vi "Autonomous Independent.vi"() -> ()   [LabVIEW 2014]
doc: "This VI is called when autonomous begins, and will automatically be terminated when autonomous ends. You can carry out timed or sensor driven robot movement independently without needing to return to the caller."
uses:
  <vilib>/ActorFramework/Message Enqueuer/Message Priority.ctl
  Robot Actor Framework/System Actor/System Actor Messages/Trace Msg/Trace Msg.lvclass/Trace Msg.ctl
  <vilib>/ActorFramework/Message Enqueuer/Message Enqueuer.lvclass/Message Enqueuer.ctl
  <vilib>/ActorFramework/Message Enqueuer/Enqueue.vi
  <vilib>/Utility/config.llb/Read Key (Boolean).vi
  Robot Global Data.vi
  <vilib>/Utility/config.llb/Read Key (U32).vi
  <vilib>/Utility/config.llb/Read Key (Double).vi
  <vilib>/ActorFramework/Message Priority Queue/Priority Enqueue.vi
  Robot/Forward Drive/Forward Drive Messages/Set Percentage Msg/Set Percentage Msg.lvclass
  Robot Actor Framework/System Actor/System Actor Messages/Trace Msg/Trace Msg.lvclass
  <vilib>/Utility/config.llb/NI_LVConfig.lvlib
  <vilib>/ActorFramework/Message Enqueuer/Message Enqueuer.lvclass
panel:
  in  "Time(ms)":u32=2500
  in  "Rate(Percentage)":dbl=-1.0 min=-1.0 max=1.0
  # "Be sure to right-click and choose Data Operations>>Make Current Value default if you want to save the array values with the VI"
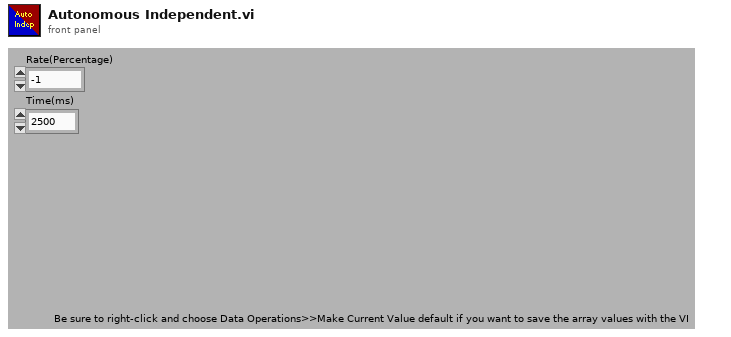
[diagram p1: front panel]
types:
  T1 = typedef "Actor Framework.lvlib/Message Enqueuer.lvclass/Message Priority.ctl" = enum16{"Low", "Normal", "High"}
  T2 = enum16{"Critical", "Error", "Warning", "Informational", "Debug"}
  T3 = typedef "NI_LVConfig.lvlib/Config Data RefNum.ctl" = refnum<k1>
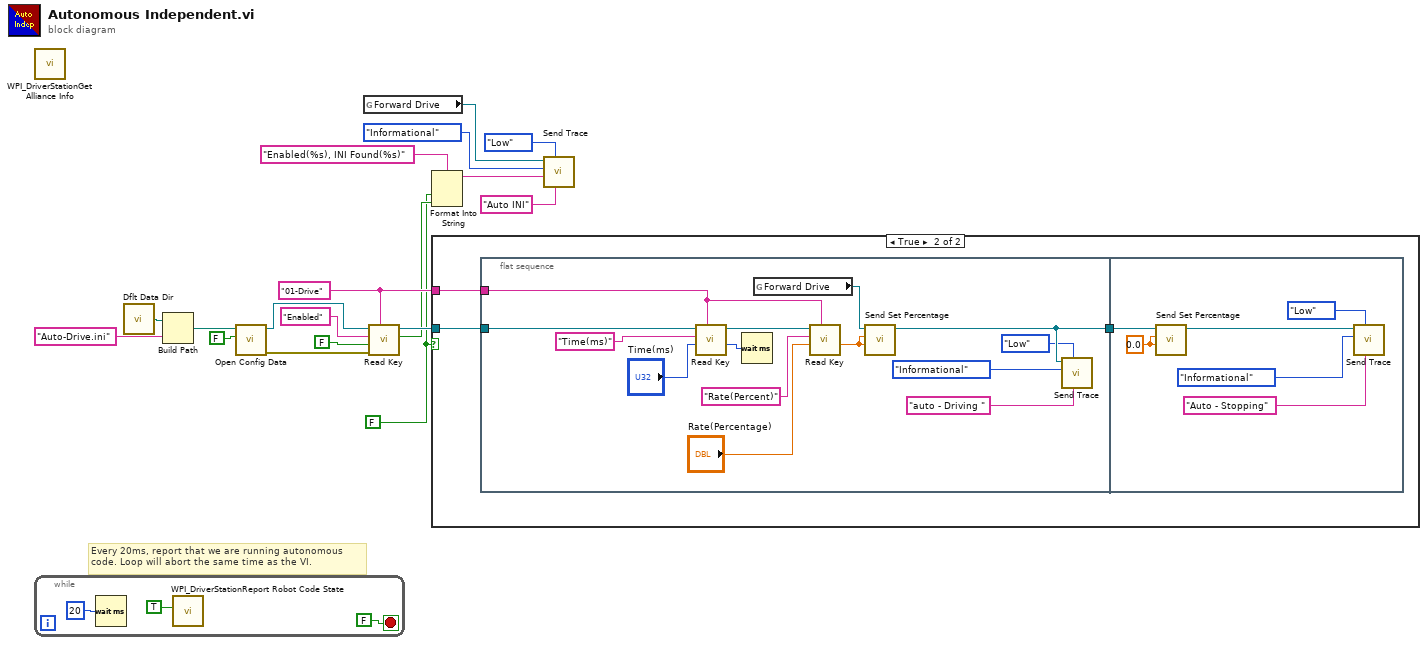
[diagram p0: block diagram]
diagram:
  w1 = FALSE
  w12 = "01-Drive" ("section")
  # "Every 20ms, report that we are running autonomous\ncode. Loop will abort the same time as the VI."
  n1 = call <vilib>:"WPI_DriverStationGet Alliance Info.vi"() -> ()  [unwired: 12 out]
  n2 = while {
    stop <- FALSE stop-if-true
    n3 = Wait (ms)(milliseconds to wait=u32 20) -> ()  [unwired: 1 out]
    n4 = call <vilib>:"WPI_DriverStationReport Robot Code State.vi"("Autonomous"=TRUE) -> ()  [unwired: 10 in, 1 out]
  }
  n5 = call <vilib>:"Dflt Data Dir.vi"() -> ("App:Default Data Directory"=w16:path)
  n6 = Build Path(base path=w16, name or relative path="Auto-Drive.ini" ("text")) -> (appended path=w15:path)
  n7 = call <vilib>:"Open Config Data.vi"("create file if necessary (T)"=FALSE, "configuration file path"=w15) -> ("error out"=w9:errorcluster, "refnum"=w14:T3)  [unwired: 7 in, 1 out]
  n8 = global read "Robot Global Data.vi" "Forward Drive"() -> (w8:refnum<class "Message Enqueuer.lvclass">)
  n9 = call-poly <vilib>:"Read Key.vi"("section"=w12, "error in (no error)"=w9, "default value"=FALSE, "key"="Enabled", "refnum"=w14) -> ("found?"=w2:bool, "refnum out"=w13:T3)  [unwired: 3 in, 2 out]
  n10 = Format Into String(format string="Enabled(%s), INI Found(%s)", w1, w2) -> (resulting string=w4:string)  [unwired: 2 in, 1 out]
  n11 = case shown="True" w1 {
    tunnel: w13 -> [_ w23]
    tunnel: w12 -> [_ w22]
    frame False {
    }
    frame True {
      n12 = flat-sequence {
        tunnel: [w28] -> w24
        tunnel: w23 -> [w37]
        tunnel: w22 -> [w29]
        tunnel: w24 -> [w43]
        frame #0 {
          n13 = call-poly <vilib>:"Read Key.vi"("section"=w29, "default value"="Time(ms)", "key"="Time(ms)", "refnum"=w37) -> ("value"=w35:u32, "refnum out"=w33:T3)  [unwired: 4 in, 2 out]
          n14 = Wait (ms)(milliseconds to wait=w35) -> ()  [unwired: 1 out]
          n15 = global read "Robot Global Data.vi" "Forward Drive"() -> (w38:refnum<class "Message Enqueuer.lvclass">)
          n16 = call-poly <vilib>:"Read Key.vi"("section"=w29, "default value"="Rate(Percentage)", "key"="Rate(Percent)", "refnum"=w33) -> ("value"=w30:dbl)  [unwired: 4 in, 3 out]
          n17 = call "Send Set Percentage.vi"("Right Percentage"=w30, "Left Percentage"=w30, "Message Enqueuer"=w38) -> ("Message Enqueuer out"=w28:refnum<class "Message Enqueuer.lvclass">)  [unwired: 7 in, 1 out]
          n18 = call "Send Trace.vi"("System Action"="auto - Driving " ("System Message"), "Message Priority (Normal)"=Message_Priority."Low", "Trace Level"=T2."Informational", "Message Enqueuer"=w28) -> ()  [unwired: 6 in, 2 out]
        }
        frame #1 {
          w44 = 0.0 ("Left Percentage")
          n19 = call "Send Set Percentage.vi"("Right Percentage"=w44, "Left Percentage"=w44, "Message Enqueuer"=w43) -> ("Message Enqueuer out"=w42:refnum<class "Message Enqueuer.lvclass">)  [unwired: 7 in, 1 out]
          n20 = call "Send Trace.vi"("System Action"="Auto - Stopping" ("System Message"), "Message Priority (Normal)"=Message_Priority."Low", "Trace Level"=T2."Informational", "Message Enqueuer"=w42) -> ()  [unwired: 6 in, 2 out]
        }
      }
    }
  }
  n21 = call "Send Trace.vi"("System Action"="Auto INI", "Message Priority (Normal)"=Message_Priority."Low", "System Message"=w4, "Trace Level"=T2."Informational", "Message Enqueuer"=w8) -> ()  [unwired: 5 in, 2 out]
